vi "GlobalClassRefs.vi"() -> ()   [LabVIEW 2014]
uses:
  DBAL/DBAL.lvclass
  FAMM/FAMM.lvclass
  AVPP/AVPP.lvclass
  HISW/HISW.lvclass
panel:
  out "HISW_class":refnum<data-value>
  out "AVPP_class":refnum<data-value>
  out "FAMM_class":refnum<data-value>
  out "DBAL_class":refnum<data-value>
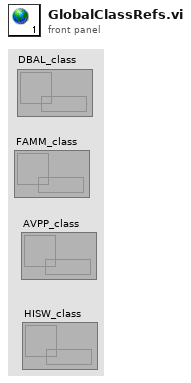
[diagram p1: front panel]
diagram:
